vi "载波.vi"(1 "相位输入":dbl, 2 "载频":dbl, 3 "采样率":dbl, 4 "采样点数":i32=128 caption="采样点数N") -> (0 "载波信号波形":dbl[](array[numeric]) caption="正弦信号")   [LabVIEW 2013]
uses:
  <vilib>/Analysis/NI_AALBase.lvlib
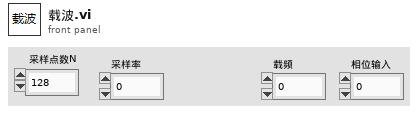
[diagram p1: front panel]
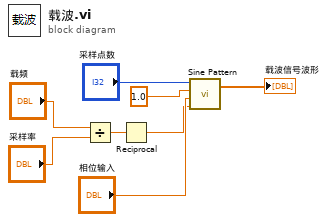
[diagram p0: block diagram]
diagram:
  n1 = Divide(x="载频", y="采样率") -> (x/y=w1:dbl)
  n2 = Reciprocal(x=w1) -> (1/x=w2:dbl)
  n3 = call <vilib>:"Sine Pattern.vi"("cycles"=w2, "phase(degrees)"="相位输入", "amplitude"=1.0, "samples"="采样点数") -> ("Sinusoidal Pattern"=→"载波信号波形":dbl[])  [unwired: 1 out]
